vi "GetError.vi"(8 "error in (no error)":errorcluster, 11 "String in":string) -> (3 "String out":string)   [LabVIEW 2012]
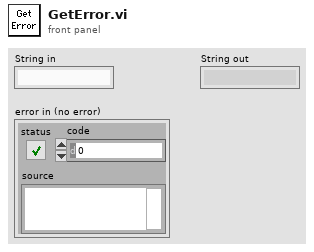
[diagram p1: front panel]
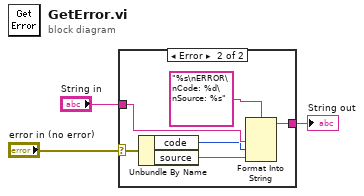
[diagram p0: block diagram]
diagram:
  n1 = case shown="Error" "error in (no error)" {
    selector: "error in (no error)" -> [_ w9]
    tunnel: "String in" -> [w4 w10]
    tunnel: [w4 w5] -> w3
    frame No Error {
    }
    frame Error {
      n2 = Unbundle By Name(w9) -> ("code"=w8:i32, "source"=w7:string)
      n3 = Format Into String(format string="%s\nERROR\nCode: %d\nSource: %s", w10, w8, w7) -> (resulting string=w5:string)  [unwired: 2 in, 1 out]
    }
  }
  "String out" <- w3
